vi "FPGA Main R2 with filter AB JC.vi"() -> ()   [LabVIEW 2018]
uses:
  <vilib>/rvi/Emulation/niFpgaGetClockAttributes.vi
  <vilib>/rvi/Emulation/niFpgaSctlEmulationGetInTimedLoop.vi
  <vilib>/rvi/Emulation/niFpgaEmulationReportErrorSimple.vi
  <vilib>/rvi/eio/common/nirviEmuTemplateMethod_errors.vi
  <vilib>/rvi/Emulation/niFpgaProcessEmulError.vi
  <vilib>/rvi/interface/RandomDataEmulation/niFpgaRandomDataHandleErrors.vi
  <vilib>/rvi/Emulation/niFpgaCriticalErrorInLSC.vi
  <vilib>/rvi/Analysis/control/PID/SubVIs/niFpgaPID_PIWrapper.vi
  <vilib>/eio/EIONode/EIONode.xnode
  <vilib>/rvi/Analysis/measure/butterworth/XNode/niFpgaButterworthFilter.xnode
  <vilib>/rvi/DataTransferAndStorage/Container/XNode/niFpgaContainer.xnode
  <vilib>/rvi/interface/RandomDataEmulation/nirviRandomDataFpgaReadWriteTemplate.vi
panel:
  in  "Manual/PID":bool
  out "PID Error (V)":sgl
  out "PID Output (V)":u16
  in  "Output Limits":cluster{"Vmax":sgl, "Vmin":sgl}
  in  "PID Gains":cluster{"Kp":sgl, "Ki":sgl}
  out "Capacitance\nProbe (V)":u16
  out "Coil Back \nEMF (V)":u16
  in  "Control Loop \nRate (uSec)":u32
  in  "Sensor Loop \nRate (uSec)":u32
  in  "VC Command (V)":u16
  in  "Amplifier On/Off":bool
  # "Controls"
  # "PID Settings"
  # "Sensors"
  # "Loop Rates"
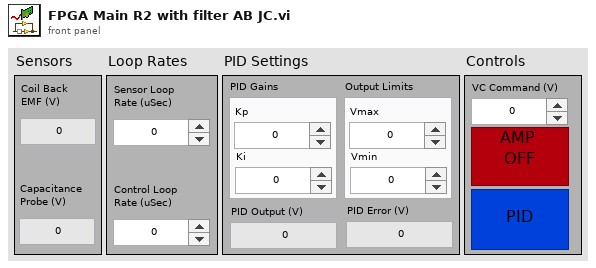
[diagram p1: front panel]
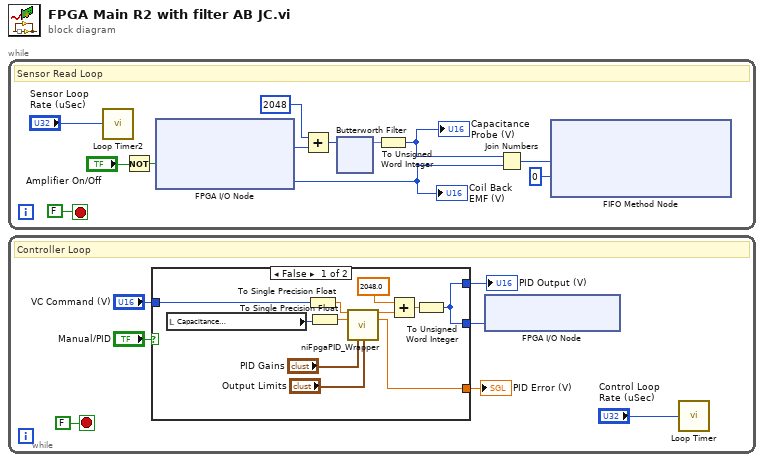
[diagram p0: block diagram]
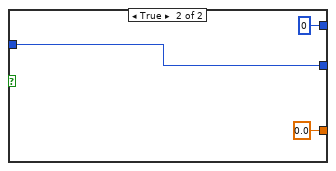
[diagram p2: hidden frame]
diagram:
  n1 = while {
    stop <- FALSE stop-if-true
    # "Sensor Read Loop"
    n2 = call "Loop Timer2"("Count(uSec)"="Sensor Loop \nRate (uSec)") -> ()  [unwired: 1 out]
    n3 = Not(x="Amplifier On/Off") -> (.not. x?=w4:bool)
    n4 = xnode "FPGA I/O Node"("ConnectorA/DIO9"=w4) -> ("ConnectorC/AI0"=w12:i16, "ConnectorA/AI1"=w8:u16)  [unwired: 3 in, 3 out]
    "Coil Back \nEMF (V)" <- w8
    n5 = Add(x=i16 2048, y=w12) -> (x+y=w3:i16)
    n6 = xnode "Butterworth Filter"("input data"=w3) -> ("output data"=w2:fxp<+/-,20,20>)  [unwired: 2 in]
    n7 = To Unsigned Word Integer(number=w2) -> (unsigned 16bit integer=w1:u16)
    "Capacitance\nProbe (V)" <- w1
    n8 = Join Numbers(hi=w1, lo=w8) -> ((hi.lo)=w9:u32)
    n9 = xnode ("FIFO Method Node")("Element"=w9, "Timeout"=0) -> ()  [unwired: 1 in, 2 out]
  }
  n10 = while {
    stop <- FALSE stop-if-true
    # "Controller Loop"
    n11 = case shown="False" "Manual/PID" {
      tunnel: "VC Command (V)" -> [w37 w39]
      tunnel: [w28 u16 0] -> w25
      tunnel: [w31 sgl 0.0 ("error")] -> w24
      tunnel: [w28 w39] -> w22
      frame False {
        n12 = local read "Capacitance\nProbe (V)"() -> (w35:u16)
        n13 = To Single Precision Float(number=w37) -> (single precision float=w36:sgl)
        n14 = To Single Precision Float(number=w35) -> (single precision float=w38:sgl)
        n15 = call-poly <vilib>:"niFpgaPID_Wrapper.vi"("setpoint"=w36, "process variable"=w38, "gains"="PID Gains", "output range"="Output Limits") -> ("output"=w30:sgl, "error"=w31:sgl)  [unwired: 9 in, 1 out]
        n16 = Add(x=sgl 2048.0, y=w30) -> (x+y=w32:sgl)
        n17 = To Unsigned Word Integer(number=w32) -> (unsigned 16bit integer=w28:u16)
      }
      frame True {
      }
    }
    "PID Output (V)" <- w25
    "PID Error (V)" <- w24
    n18 = xnode "FPGA I/O Node"("ConnectorA/AO1"=w22) -> ()  [unwired: 1 in, 1 out]
    n19 = call "Loop Timer"("Count(uSec)"="Control Loop \nRate (uSec)") -> ()  [unwired: 1 out]
  }
